vi "Initialize Light Stack.vi"(8 "error in (no error)":errorcluster, 11 "DigitalIO in":refnum<class "DigitalIO.lvclass">) -> (0 "error out":errorcluster, 3 "DigitalIO out":refnum<class "DigitalIO.lvclass">)   [LabVIEW 2018, in "DigitalIO.lvlib" / "DigitalIO.lvclass"]
uses:
  DigitalIO.lvclass
  DigitalIO.lvclass/DigitalIO.ctl
  PPLs/PLC/Light Stack.lvlibp/Light Stack.lvclass
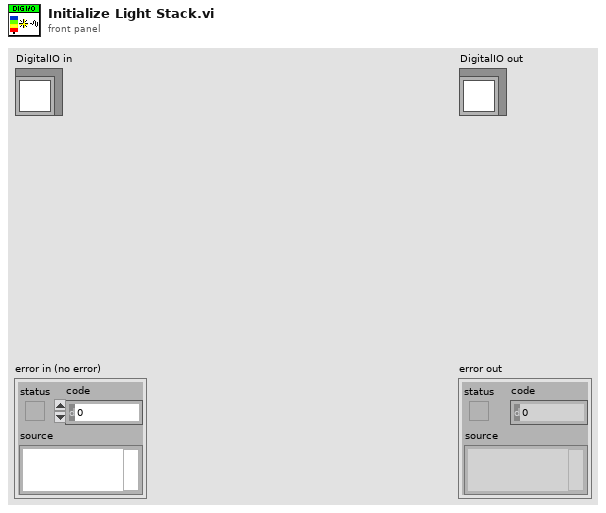
[diagram p1: front panel]
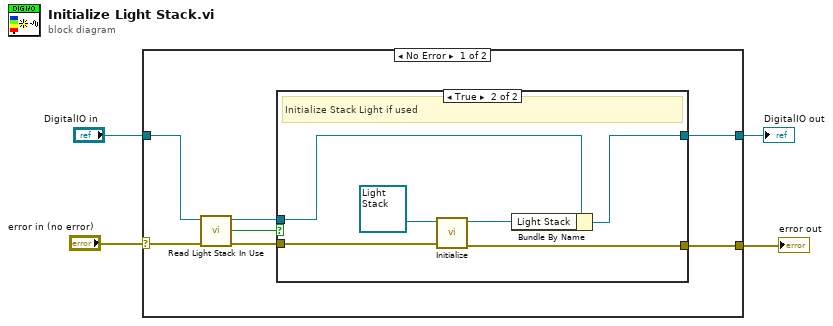
[diagram p0: block diagram]
diagram:
  n1 = case shown="No Error" "error in (no error)" {
    selector: "error in (no error)" -> [w10 w21]
    tunnel: [w5 w21] -> w3
    tunnel: [w6 w20] -> w1
    tunnel: "DigitalIO in" -> [w11 w20]
    frame No Error {
      n2 = call "Read Light Stack In Use.vi"("error in (no error)"=w10, "DigitalIO in"=w11) -> ("error out"=w8:errorcluster, "Light Stack In Use?"=w9:bool, "DigitalIO out"=w7:refnum<class "DigitalIO.lvclass">)  [unwired: 7 in]
      n3 = case shown="True" w9 {
        tunnel: w8 -> [w13 w18]
        tunnel: w7 -> [w12 w17]
        tunnel: [w12 w15] -> w6
        tunnel: [w13 w14] -> w5
        frame False {
        }
        frame True {
          # "Initialize Stack Light if used"
          n4 = call "Initialize.vi"("error in"=w18, "Light Stack in"=refnum<class "Light Stack.lvclass"> refnum ("Light Stack.lvlibp:Light Stack.lvclass")) -> ("error out"=w14:errorcluster, "Light Stack out"=w16:refnum<class "Light Stack.lvclass">)  [unwired: 8 in]
          n5 = Bundle By Name(cluster=w17, "Light Stack"=w16) -> (w15:refnum<class "DigitalIO.lvclass">)
        }
      }
    }
    frame Error {
    }
  }
  "error out" <- w3
  "DigitalIO out" <- w1
